vi "imageQ_dequeue.vi"(6 "timeout in ms (-1)":i32=-1, 10 "Return queue":refnum<queue>, 11 "Image Dst":T1) -> (1 "Timestamp/us":u64=2, 2 "Return queue out":refnum<queue>, 3 "Image Dst Out":T1, 4 "timed out?":bool, 5 "ROI":u64[](array[numeric]))   [LabVIEW 2010]
uses:
  <vilib>/vision/Image Controls.llb/IMAQ Image.ctl
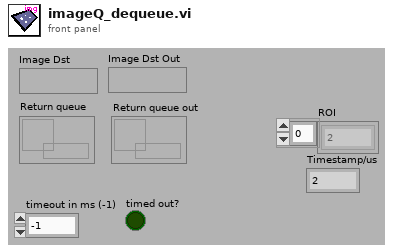
[diagram p1: front panel]
types:
  T1 = typedef "IMAQ Image.ctl" = refnum<image>
  T2 = cluster{"New Image":T1, "queue out":refnum<queue>}
  T3 = cluster{"Camera Image":T1, "ROI":u64[], "Timestamp/us":u64}
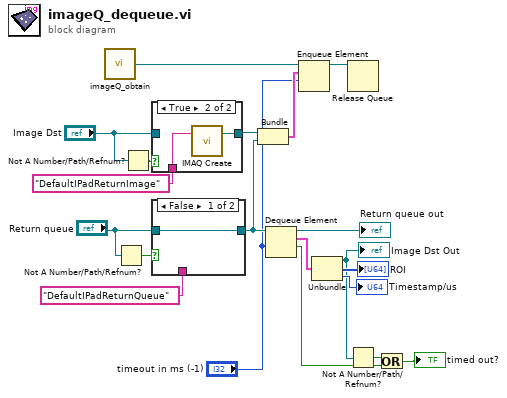
[diagram p0: block diagram]
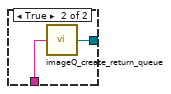
[diagram p3: hidden frame]
diagram:
  n1 = call "imageQ_obtain.vi"() -> ("queue out"=w17:refnum<queue>)
  n2 = Not A Number/Path/Refnum?(number/path/refnum="Return queue") -> (NaN/Path/Refnum?=w16:bool)
  n3 = Not A Number/Path/Refnum?(number/path/refnum="Image Dst") -> (NaN/Path/Refnum?=w13:bool)
  n4 = case shown="True" w13 {
    tunnel: "Image Dst" -> [w21 _]
    tunnel: "DefaultIPadReturnImage" -> [_ w23]
    tunnel: [w21 w22] -> w10
    frame False {
    }
    frame True {
      n5 = call "IMAQ Create"("Image Name"=w23) -> ("New Image"=w22:T1)  [unwired: 4 in, 1 out]
    }
  }
  n6 = case shown="False" w16 {
    tunnel: "Return queue" -> [w24 _]
    tunnel: [w24 w26] -> w9
    tunnel: "DefaultIPadReturnQueue" -> [_ w25]
    frame False {
    }
    frame True {
      n7 = call "imageQ_create_return_queue.vi"("Queue Name"=w25) -> ("queue out"=w26:refnum<queue>)
    }
  }
  n8 = Bundle("New Image"=w10, "queue out"=w9) -> (w8:T2)  [unwired: 1 in]
  n9 = Dequeue Element(queue=w9, timeout in ms (-1)="timeout in ms (-1)") -> (queue out=→"Return queue out":refnum<queue>, element=w20:T3, timed out?=w4:bool)  [unwired: 1 in, 1 out]
  n10 = Enqueue Element(queue=w17, element=w8, timeout in ms (-1)="timeout in ms (-1)") -> (queue out=w7:refnum<queue>)  [unwired: 1 in, 2 out]
  n11 = Unbundle(w20) -> ("Camera Image"=w3:T1, "ROI"=→"ROI":u64[], "Timestamp/us"=→"Timestamp/us":u64)
  "Image Dst Out" <- w3
  n12 = Release Queue(queue=w7) -> ()  [unwired: 2 in, 3 out]
  n13 = Not A Number/Path/Refnum?(number/path/refnum=w3) -> (NaN/Path/Refnum?=w1:bool)
  n14 = Or(x=w1, y=w4) -> (x .or. y?=→"timed out?":bool)
